vi "Test.vi"() -> ()   [LabVIEW 2020]
uses:
  Com/SECS Communication/HSMS Class/HSMS State.ctl
  Com/SECS Communication/HSMS Class/Role.ctl
  Com/SECS Communication/HSMS Class/HSMS Class.lvclass/HSMS Class.ctl
  Com/SECS Communication/S6 Message Class/S6 Message Class.lvclass
  D:/Dropbox/SECS/SECS_GEM v1.1.0/Com/SECS Communication/SECS-II Class/SECS-II Class.lvclass
  Com/SECS Communication/S1 Message Class/S1 Message Class.lvclass
  Com/SECS Communication/S2 Message Class/S2 Message Class.lvclass
  Com/SECS Communication/S5 Message Class/S5 Message Class.lvclass
  Com/SECS Communication/HSMS Class/Notifier Data.ctl
  Com/SECS Communication/HSMS Class/Notifier Type.ctl
  Com/SECS Communication/HSMS Class/Read HSMS State.vi
  Com/SECS Communication/HSMS Class/Write Session ID.vi
  Com/SECS Communication/HSMS Class/Write Log Path.vi
  Com/SECS Communication/HSMS Class/Read Recive User Event.vi
  Com/SECS Communication/HSMS Class/Read Notifier User Event.vi
  Com/SECS Communication/HSMS Class/Write T3(Reply Timeout).vi
  Com/SECS Communication/SECS-II Class/SECS-II Class.lvclass
  Com/SECS Communication/HSMS Class/HSMS Class.lvclass
panel:
  out "Stop":bool=TRUE
  in  "Test Count":i32
  in  "Random Test":bool
  in  "Message":T1(ring)
  out "Notifier Data":string
  in  "Send":bool
  out "HSMS State":T2=enum."Stop"
  in  "Stop HSMS":bool
  in  "Start HSMS":bool
  in  "IP Adrress":string="127.0.0.1"
  in  "Port":u16=5000
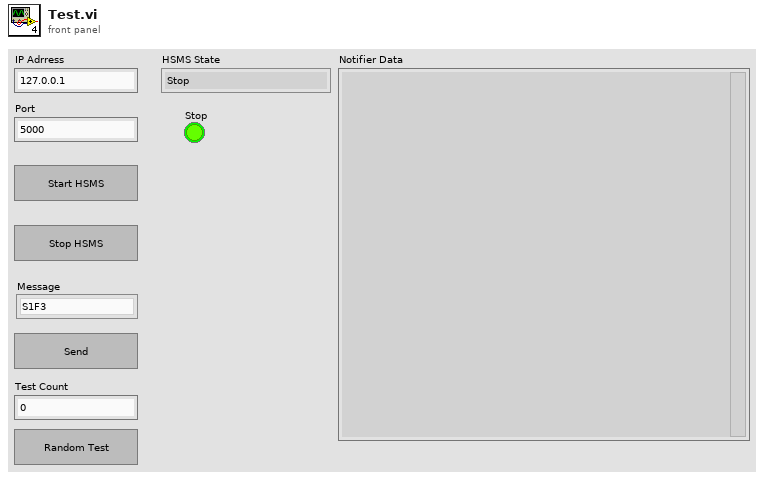
[diagram p1: front panel]
types:
  T1 = enum16{"S1F3", "S1F13", "S1F17", "S2F31", "S2F33", "S2F35", "S2F37", "S5F3", "S5F5", "S6F1"}
  T2 = typedef "SECS Communication.lvlib/HSMS Class.lvclass/HSMS State.ctl" = enum16{"[TCP/IP]Not Connect", "[HSMS]Not Selected", "[HSMS]Selected", "Stop"}
  T3 = typedef "SECS Communication.lvlib/HSMS Class.lvclass/Role.ctl" = enum16{"Passive", "Active"}
  T4 = typedef "SECS Communication.lvlib/HSMS Class.lvclass/Notifier Data.ctl" = cluster{"Notifier Type":T5, "Data":variant, "Time":timestamp}
  T5 = typedef "SECS Communication.lvlib/HSMS Class.lvclass/Notifier Type.ctl" = enum16{"TCPIP Connect", "TCPIP Disconnect", "Receive Message", "Send Message", "T3 Timeout", "T6 Timeout", "T7 Timeout", "Error", "Stop"}
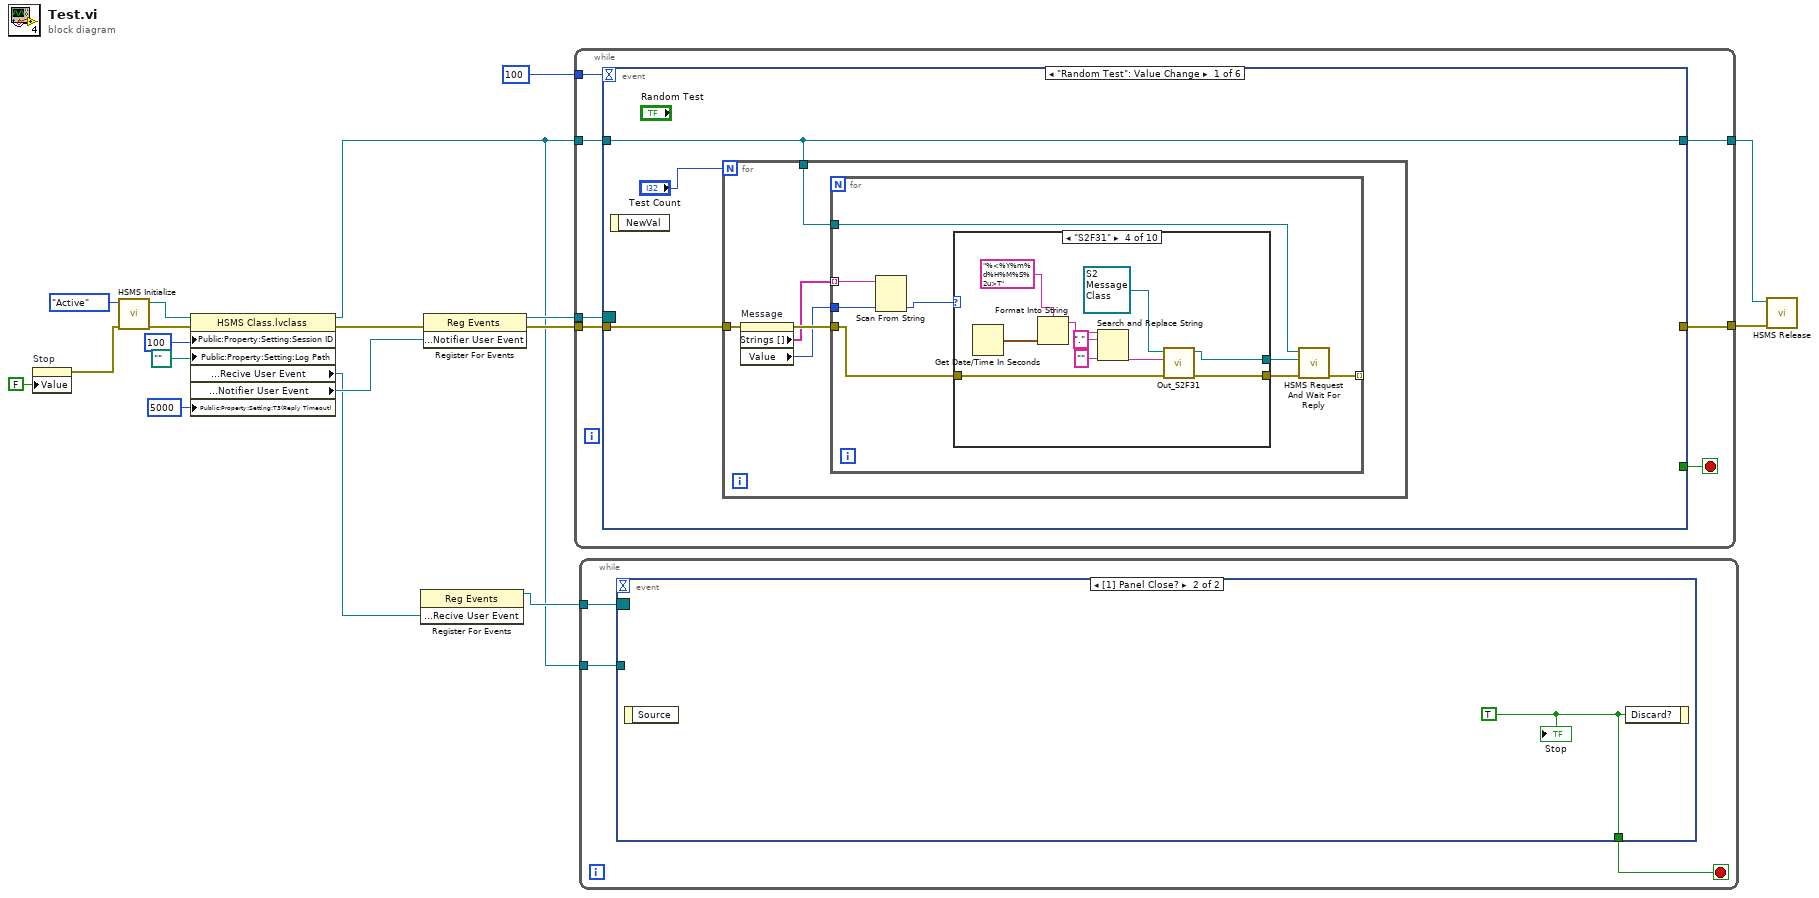
[diagram p0: block diagram]
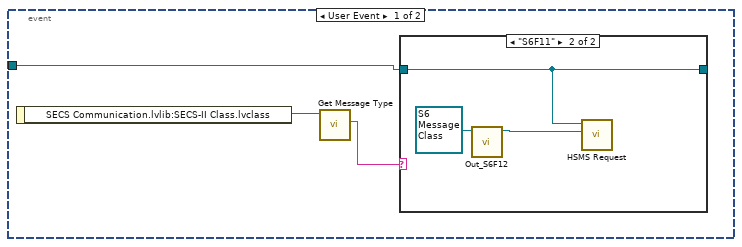
[diagram p2: hidden frame]
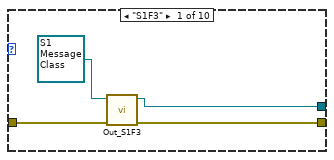
[diagram p4: hidden frame]
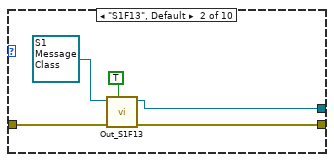
[diagram p5: hidden frame]
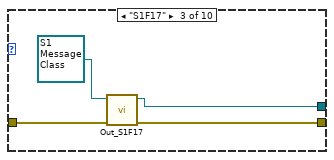
[diagram p6: hidden frame]
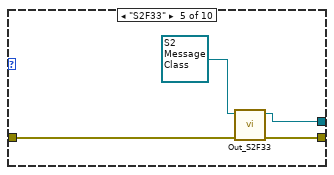
[diagram p7: hidden frame]
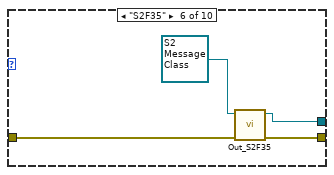
[diagram p8: hidden frame]
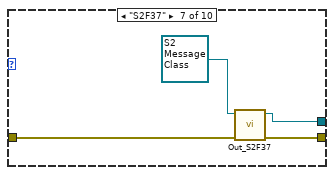
[diagram p9: hidden frame]
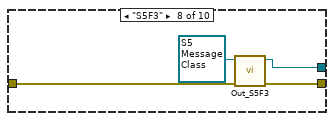
[diagram p10: hidden frame]
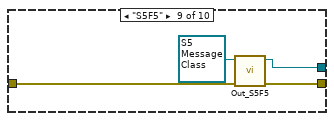
[diagram p11: hidden frame]
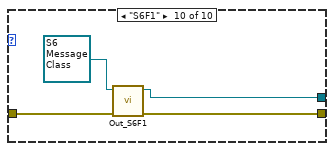
[diagram p12: hidden frame]
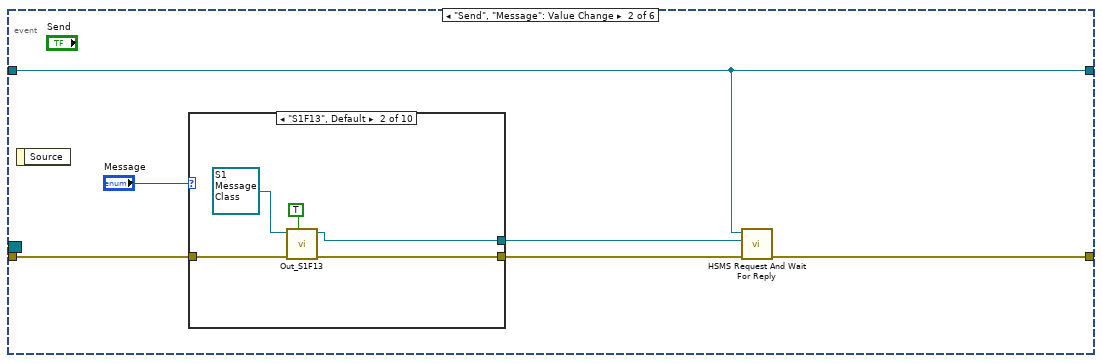
[diagram p13: hidden frame]
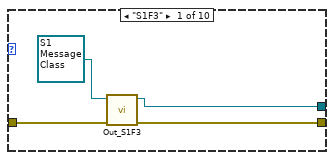
[diagram p14: hidden frame]
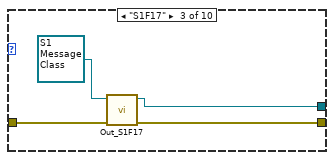
[diagram p15: hidden frame]
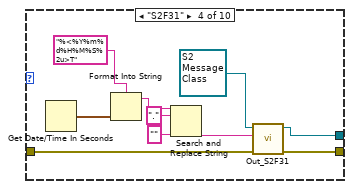
[diagram p16: hidden frame]
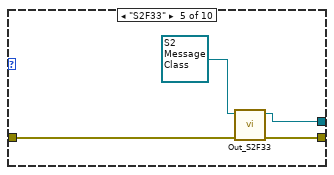
[diagram p17: hidden frame]
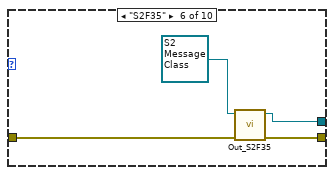
[diagram p18: hidden frame]
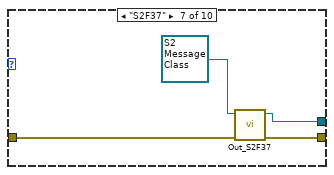
[diagram p19: hidden frame]
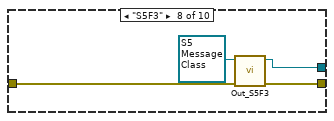
[diagram p20: hidden frame]
diagram:
  n1 = property on="Stop" class="Bool (strict)"("Value"=FALSE ("Stop")) -> (error out=w3:errorcluster)  [unwired: 2 in, 1 out]
  n2 = call "HSMS Initialize.vi"("error in (no error)"=w3, "Role"=Role."Active") -> ("error out"=w10:errorcluster, "HSMS Class out"=w9:refnum<class "HSMS Class.lvclass">)  [unwired: 8 in]
  n3 = property class="HSMS Class.lvclass"(reference=w9, error in=w10, "Public:Property:Setting:Session ID"=u16 100 ("Session ID"), "Public:Property:Setting:Log Path"=path "" ("Log Path"), "Public:Property:Setting:T3(Reply Timeout)"=5000 ("Setting:T3(Reply Timeout)")) -> (reference out=w4:refnum<class "HSMS Class.lvclass">, error out=w14:errorcluster, "Public:Property:User Event:Recive User Event"=w6:refnum<user-event>, "Public:Property:User Event:Notifier User Event"=w7:refnum<user-event>)
  n4 = register-events(w6) -> (reference out=w5:refnum<event-registration>)  [unwired: 2 in, 1 out]
  n5 = register-events(error in=w14, w7) -> (reference out=w12:refnum<event-registration>, error out=w13:errorcluster)  [unwired: 1 in]
  n6 = while {
    tunnel: w4 -> [w25]
    tunnel: [w24] -> w17
    tunnel: [w23] -> w16
    tunnel: 100 -> [w21]
    tunnel: w13 -> [w20]
    tunnel: w12 -> [w19]
    stop <- w22 stop-if-true
    n7 = event shown="[0] \"Random Test\": Value Change" {
      selector: w19 -> [_ _ _ _ _ _]
      dyn-events: _ -> [_ _ _ _ _ _]
      timeout: w21 -> [_ _ _ _ _ _]
      tunnel: w25 -> [w27 w91 w145 w151 w156 w159]
      tunnel: [_ w90 w143 w149 w155 w158] -> w24
      tunnel: [w27 w91 w144 w150 w156 w159] -> w23
      tunnel: [_ _ _ _ w152 _] -> w22
      tunnel: w20 -> [w28 w94 w142 w148 w153 w161]
      event "Random Test": Value Change {
        n8 = event-data() -> ()  [unwired: 1 in, 1 out]
        n9 = for {
          N: "Test Count" -> [_]
          tunnel: w28 -> [w33]
          tunnel: w27 -> [w29]
          n10 = property on="Message" class="Enum (strict)"(error in=w33) -> (error out=w32:errorcluster, "Strings []"=w31:string[], "Value"=w30:T1)  [unwired: 1 in, 1 out]
          n11 = for {
            tunnel: w32 -> [w37]
            tunnel: w31 -> [w41] mode=indexing
            tunnel: w30 -> [w40]
            tunnel: w29 -> [w38]
            tunnel: [w34] -> _ mode=indexing
            n12 = Scan From String(input string=w41, default 1=w40) -> (output 1=w36:T1)  [unwired: 3 in, 3 out]
            n13 = case shown="\"S2F31\"" w36 {
              tunnel: w37 -> [w45 w50 w54 w64 w68 w72 w76 w80 w84 w85]
              tunnel: [w44 w49 w53 w63 w67 w71 w75 w79 w83 w88] -> w39
              tunnel: [w43 w48 w52 w62 w66 w70 w74 w78 w82 w87] -> w35
              frame "S1F3" {
                n14 = call "Out_S1F3.vi"("error in (no error)"=w45, "S1 Message Class in"=refnum<class "S1 Message Class.lvclass"> refnum) -> ("error out"=w44:errorcluster, "S1 Message Class out"=w43:refnum<class "S1 Message Class.lvclass">)  [unwired: 8 in]
              }
              frame "S1F13", Default {
                n15 = call "Out_S1F13.vi"("Host"=TRUE, "error in (no error)"=w50, "S1 Message Class in"=refnum<class "S1 Message Class.lvclass"> refnum) -> ("error out"=w49:errorcluster, "S1 Message Class out"=w48:refnum<class "S1 Message Class.lvclass">)  [unwired: 7 in]
              }
              frame "S1F17" {
                n16 = call "Out_S1F17.vi"("error in (no error)"=w54, "S1 Message Class in"=refnum<class "S1 Message Class.lvclass"> refnum) -> ("error out"=w53:errorcluster, "S1 Message Class out"=w52:refnum<class "S1 Message Class.lvclass">)  [unwired: 8 in]
              }
              frame "S2F31" {
                n17 = Get Date/Time In Seconds() -> (seconds since 1Jan1904=w60:timestamp)
                n18 = Format Into String(format string="%<%Y%m%d%H%M%S%2u>T", w60) -> (resulting string=w58:string)  [unwired: 2 in, 1 out]
                n19 = Search and Replace String(input string=w58, search string=".", replace string="" ("replace string (\"\")")) -> (result string=w57:string)  [unwired: 5 in, 3 out]
                n20 = call "Out_S2F31.vi"("error in (no error)"=w64, "Time"=w57, "S2 Message Class in"=refnum<class "S2 Message Class.lvclass"> refnum) -> ("error out"=w63:errorcluster, "S2 Message Class out"=w62:refnum<class "S2 Message Class.lvclass">)  [unwired: 7 in]
              }
              frame "S2F33" {
                n21 = call "Out_S2F33.vi"("error in (no error)"=w68, "S2 Message Class in"=refnum<class "S2 Message Class.lvclass"> refnum) -> ("error out"=w67:errorcluster, "S2 Message Class out"=w66:refnum<class "S2 Message Class.lvclass">)  [unwired: 8 in]
              }
              frame "S2F35" {
                n22 = call "Out_S2F35.vi"("error in (no error)"=w72, "S2 Message Class in"=refnum<class "S2 Message Class.lvclass"> refnum) -> ("error out"=w71:errorcluster, "S2 Message Class out"=w70:refnum<class "S2 Message Class.lvclass">)  [unwired: 8 in]
              }
              frame "S2F37" {
                n23 = call "Out_S2F37.vi"("error in (no error)"=w76, "S2 Message Class in"=refnum<class "S2 Message Class.lvclass"> refnum) -> ("error out"=w75:errorcluster, "S2 Message Class out"=w74:refnum<class "S2 Message Class.lvclass">)  [unwired: 8 in]
              }
              frame "S5F3" {
                n24 = call "Out_S5F3.vi"("error in (no error)"=w80, "S5 Message Class in"=refnum<class "S5 Message Class.lvclass"> refnum) -> ("error out"=w79:errorcluster, "S5 Message Class out"=w78:refnum<class "S5 Message Class.lvclass">)  [unwired: 8 in]
              }
              frame "S5F5" {
                n25 = call "Out_S5F5.vi"("error in (no error)"=w84, "S5 Message Class in"=refnum<class "S5 Message Class.lvclass"> refnum) -> ("error out"=w83:errorcluster, "S5 Message Class out"=w82:refnum<class "S5 Message Class.lvclass">)  [unwired: 8 in]
              }
              frame "S6F1" {
                n26 = call "Out_S6F1.vi"("error in (no error)"=w85, "S6 Message Class in"=refnum<class "S6 Message Class.lvclass"> refnum ("SECS Communication.lvlib:S6 Message Class.lvclass")) -> ("error out"=w88:errorcluster, "S6 Message Class out"=w87:refnum<class "S6 Message Class.lvclass">)  [unwired: 8 in]
              }
            }
            n27 = call "HSMS Request And Wait For Reply.vi"("error in (no error)"=w39, "SECS-II Class In"=w35, "HSMS Class in"=w38) -> ("error out"=w34:errorcluster)  [unwired: 5 in, 3 out]
          }
        }
      }
      event "Send", "Message": Value Change {
        n28 = event-data() -> ()  [unwired: 1 in, 1 out]
        n29 = case shown="\"S1F13\", Default" "Message" {
          tunnel: w94 -> [w98 w103 w107 w117 w121 w125 w129 w133 w137 w138]
          tunnel: [w97 w102 w106 w116 w120 w124 w128 w132 w136 w141] -> w92
          tunnel: [w96 w101 w105 w115 w119 w123 w127 w131 w135 w140] -> w89
          frame "S1F3" {
            n30 = call "Out_S1F3.vi"("error in (no error)"=w98, "S1 Message Class in"=refnum<class "S1 Message Class.lvclass"> refnum) -> ("error out"=w97:errorcluster, "S1 Message Class out"=w96:refnum<class "S1 Message Class.lvclass">)  [unwired: 8 in]
          }
          frame "S1F13", Default {
            n31 = call "Out_S1F13.vi"("Host"=TRUE, "error in (no error)"=w103, "S1 Message Class in"=refnum<class "S1 Message Class.lvclass"> refnum) -> ("error out"=w102:errorcluster, "S1 Message Class out"=w101:refnum<class "S1 Message Class.lvclass">)  [unwired: 7 in]
          }
          frame "S1F17" {
            n32 = call "Out_S1F17.vi"("error in (no error)"=w107, "S1 Message Class in"=refnum<class "S1 Message Class.lvclass"> refnum) -> ("error out"=w106:errorcluster, "S1 Message Class out"=w105:refnum<class "S1 Message Class.lvclass">)  [unwired: 8 in]
          }
          frame "S2F31" {
            n33 = Get Date/Time In Seconds() -> (seconds since 1Jan1904=w113:timestamp)
            n34 = Format Into String(format string="%<%Y%m%d%H%M%S%2u>T", w113) -> (resulting string=w111:string)  [unwired: 2 in, 1 out]
            n35 = Search and Replace String(input string=w111, search string=".", replace string="" ("replace string (\"\")")) -> (result string=w110:string)  [unwired: 5 in, 3 out]
            n36 = call "Out_S2F31.vi"("error in (no error)"=w117, "Time"=w110, "S2 Message Class in"=refnum<class "S2 Message Class.lvclass"> refnum) -> ("error out"=w116:errorcluster, "S2 Message Class out"=w115:refnum<class "S2 Message Class.lvclass">)  [unwired: 7 in]
          }
          frame "S2F33" {
            n37 = call "Out_S2F33.vi"("error in (no error)"=w121, "S2 Message Class in"=refnum<class "S2 Message Class.lvclass"> refnum) -> ("error out"=w120:errorcluster, "S2 Message Class out"=w119:refnum<class "S2 Message Class.lvclass">)  [unwired: 8 in]
          }
          frame "S2F35" {
            n38 = call "Out_S2F35.vi"("error in (no error)"=w125, "S2 Message Class in"=refnum<class "S2 Message Class.lvclass"> refnum) -> ("error out"=w124:errorcluster, "S2 Message Class out"=w123:refnum<class "S2 Message Class.lvclass">)  [unwired: 8 in]
          }
          frame "S2F37" {
            n39 = call "Out_S2F37.vi"("error in (no error)"=w129, "S2 Message Class in"=refnum<class "S2 Message Class.lvclass"> refnum) -> ("error out"=w128:errorcluster, "S2 Message Class out"=w127:refnum<class "S2 Message Class.lvclass">)  [unwired: 8 in]
          }
          frame "S5F3" {
            n40 = call "Out_S5F3.vi"("error in (no error)"=w133, "S5 Message Class in"=refnum<class "S5 Message Class.lvclass"> refnum) -> ("error out"=w132:errorcluster, "S5 Message Class out"=w131:refnum<class "S5 Message Class.lvclass">)  [unwired: 8 in]
          }
          frame "S5F5" {
            n41 = call "Out_S5F5.vi"("error in (no error)"=w137, "S5 Message Class in"=refnum<class "S5 Message Class.lvclass"> refnum) -> ("error out"=w136:errorcluster, "S5 Message Class out"=w135:refnum<class "S5 Message Class.lvclass">)  [unwired: 8 in]
          }
          frame "S6F1" {
            n42 = call "Out_S6F1.vi"("error in (no error)"=w138, "S6 Message Class in"=refnum<class "S6 Message Class.lvclass"> refnum ("SECS Communication.lvlib:S6 Message Class.lvclass")) -> ("error out"=w141:errorcluster, "S6 Message Class out"=w140:refnum<class "S6 Message Class.lvclass">)  [unwired: 8 in]
          }
        }
        n43 = call "HSMS Request And Wait For Reply.vi"("error in (no error)"=w92, "SECS-II Class In"=w89, "HSMS Class in"=w91) -> ("error out"=w90:errorcluster)  [unwired: 5 in, 3 out]
      }
      event "Stop HSMS": Value Change {
        n44 = event-data() -> ()  [unwired: 1 in, 1 out]
        n45 = call "HSMS Stop.vi"("error in (no error)"=w142, "HSMS Class in"=w145) -> ("error out"=w143:errorcluster, "HSMS Class out"=w144:refnum<class "HSMS Class.lvclass">)  [unwired: 8 in]
      }
      event "Start HSMS": Value Change {
        n46 = event-data() -> ()  [unwired: 1 in, 1 out]
        n47 = call "HSMS Start.vi"("error in (no error)"=w148, "Port"="Port", "IP Adrress"="IP Adrress", "HSMS Class in"=w151) -> ("error out"=w149:errorcluster, "HSMS Class out"=w150:refnum<class "HSMS Class.lvclass">)  [unwired: 6 in]
      }
      event Timeout {
        n48 = event-data() -> ()  [unwired: 1 in, 1 out]
        n49 = property class="HSMS Class.lvclass"(reference=w156, error in=w153) -> (error out=w155:errorcluster, "Public:Property:HSMS State"=→"HSMS State":T2)  [unwired: 1 out]
        n50 = local read "Stop"() -> (w152:bool)
      }
      event User Event {
        n51 = event-data() -> ("Notifier Type"=w165:T5, "Data"=w164:variant, "Time"=w163:timestamp)  [unwired: 1 in]
        n52 = Bundle By Name(cluster=T4 {"Notifier Type"=enum."Receive Message", "Data"=variant, "Time"=timestamp(0 s since 1904-01-01)} ("Notifier Data"), "Notifier Type"=w165, "Data"=w164, "Time"=w163) -> (w160:T4)
        n53 = call "HSMS Notifier Data To String.vi"("error in (no error)"=w161, "Notifier Data"=w160) -> ("error out"=w158:errorcluster, "String"=→"Notifier Data":string)  [unwired: 8 in]
      }
    }
  }
  n54 = while {
    tunnel: w5 -> [w168]
    tunnel: w4 -> [w167]
    stop <- w166 stop-if-true
    n55 = event shown="[1] Panel Close?" {
      selector: w168 -> [_ _]
      dyn-events: _ -> [_ _]
      timeout: _ -> [_ _]
      tunnel: w167 -> [w169 _]
      tunnel: [_ w176] -> w166
      event User Event {
        n56 = event-data() -> ("SECS Communication.lvlib:SECS-II Class.lvclass"=w171:refnum<class "SECS-II Class.lvclass">)  [unwired: 1 in]
        n57 = call "Get Message Type.vi"("SECS-II Class in"=w171) -> ("Message Type"=w170:string)  [unwired: 7 in, 3 out]
        n58 = case shown="\"S6F11\"" w170 {
          tunnel: w169 -> [w172 w173]
          tunnel: [w172 w173] -> _
          frame Default {
          }
          frame "S6F11" {
            n59 = call "Out_S6F12.vi"("S6 Message Class in"=refnum<class "S6 Message Class.lvclass"> refnum) -> ("S6 Message Class out"=w174:refnum<class "S6 Message Class.lvclass">)  [unwired: 9 in, 1 out]
            n60 = call "HSMS Request.vi"("SECS-II Class In"=w174, "HSMS Class in"=w173) -> ()  [unwired: 8 in, 2 out]
          }
        }
      }
      event Panel Close? {
        w176 = TRUE ("Discard?")
        n61 = event-data() -> ()  [unwired: 1 in, 1 out]
        n62 = event-data("Discard?"=w176) -> ()  [unwired: 1 in, 1 out]
        "Stop" <- w176
      }
    }
  }
  n63 = call "HSMS Release.vi"("error in (no error)"=w17, "HSMS Class in"=w16) -> ()  [unwired: 9 in, 1 out]
